vi "initializeDefaultFont.vi"(8 "error in (no error)":errorcluster, 11 "Heading 1 in":refnum<class "Heading 1.lvclass">) -> (0 "error out":errorcluster, 3 "Heading 1 out":refnum<class "Heading 1.lvclass">)   [LabVIEW 2020, in "Styles.lvlib" / "Heading 1.lvclass"]
uses:
  Heading 1.lvclass
  Heading/Heading.lvclass
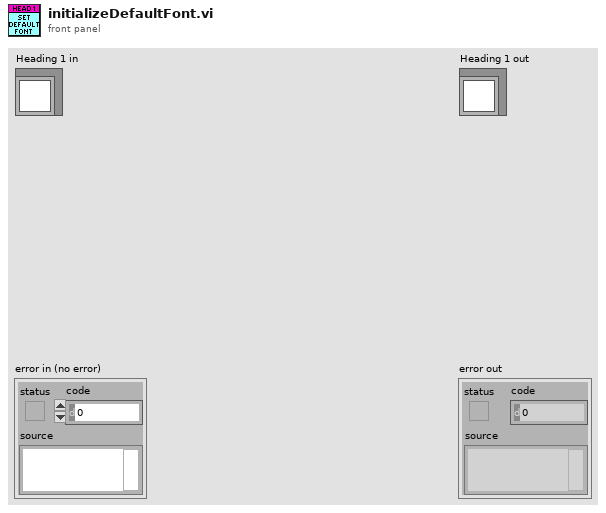
[diagram p1: front panel]
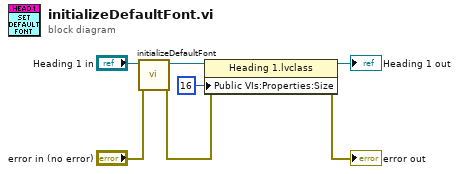
[diagram p0: block diagram]
diagram:
  n1 = call-parent "initializeDefaultFont.vi"("error in (no error)"="error in (no error)", "Heading in"="Heading 1 in") -> ("error out"=w3:errorcluster, "Heading out"=w7:refnum<class "Heading 1.lvclass">)  [unwired: 8 in]
  n2 = property class="Heading 1.lvclass"(reference=w7, error in=w3, "Public VIs:Properties:Size"=16 ("Style:Size")) -> (reference out=→"Heading 1 out":refnum<class "Heading 1.lvclass">, error out=→"error out":errorcluster)
